vi "edit.vi"(8 "error in (no error)":errorcluster, 11 "BaseM1M3Settings in":refnum<class "M1M3Settings.lvclass">) -> (0 "error out":errorcluster, 2 "cancelIsTrue out":bool, 3 "BaseM1M3Settings out":refnum<class "M1M3Settings.lvclass">)   [LabVIEW 2016, in "M1M3Settings.lvclass"]
uses:
  M1M3Settings.lvclass
  D:/Code/ts_M1M3Support/Settings/Settings/Setting.lvclass
  DataTypes/Settings/Set/HPSettings.ctl
  Settings/Setting.lvclass/Setting.ctl
  <vilib>/Utility/xml.llb/Write to XML File(string).vi
  Settings/Setting.lvclass
  DataTypes/Settings/M1M3SupportSettings.lvlib
panel:
  in  "SettingTab":enum32{"HP Settings"}(tab)
  in  "HPSettings":T1
  in  "cancelIsTrue":bool
  out "String":string
  in  "saveIsTrue":bool
  in  "Listbox":i32(listbox)
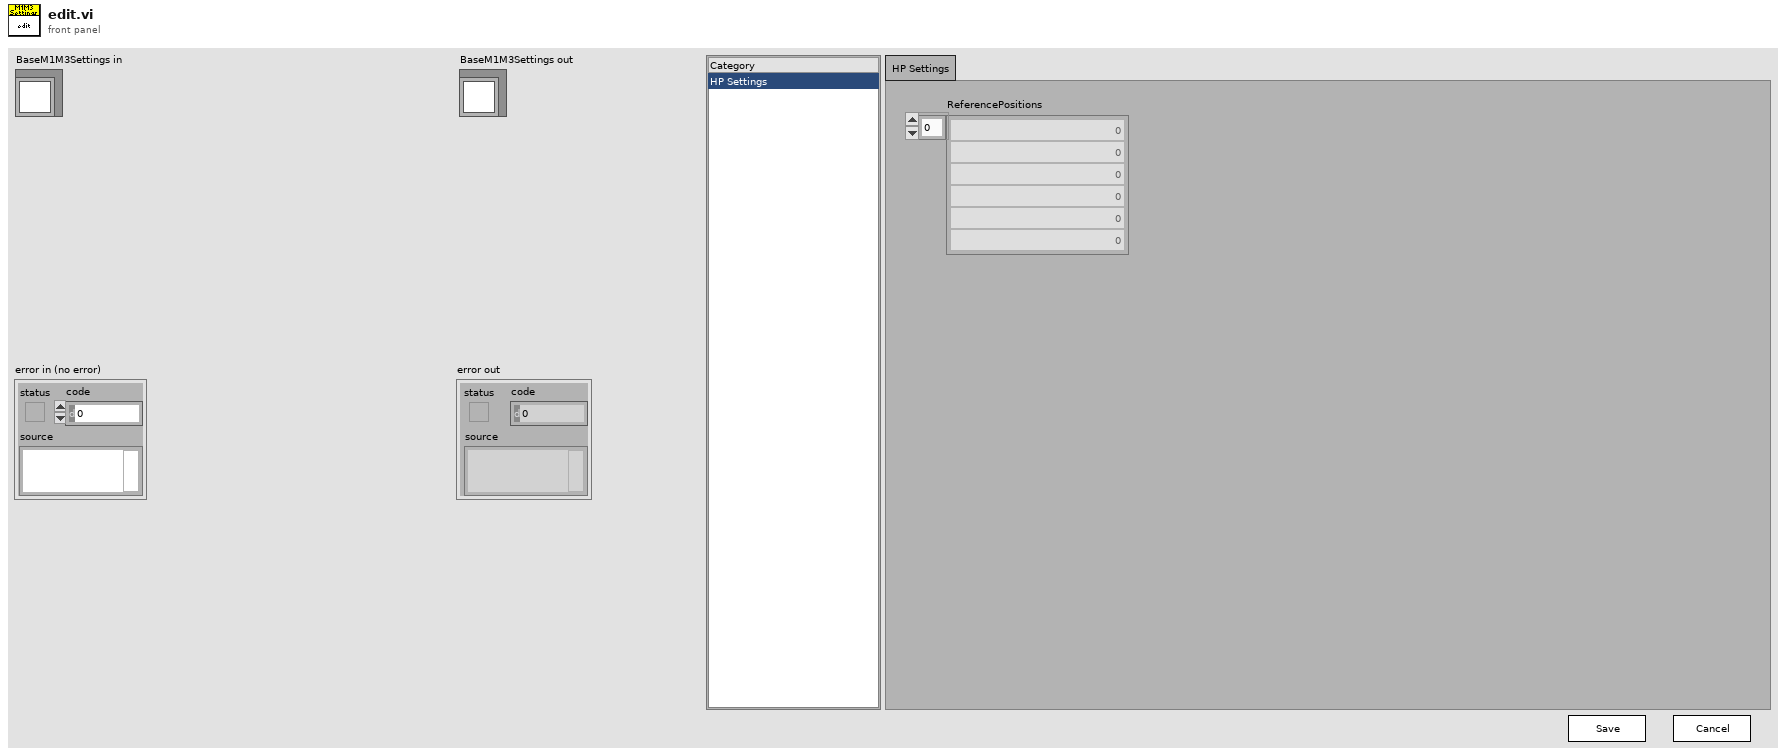
[diagram p1: front panel]
types:
  T1 = typedef "M1M3SupportSettings.lvlib/HPSettings.ctl" = cluster{"ReferencePositions":i32[]}
  T2 = enum16{"open", "replace", "create", "open or create", "replace or create", "replace or create with confirmation"}
  T3 = typedef "M1M3SupportTypes.lvlib/HPSettings.ctl" = cluster{"ReferencePositions":i32[]}
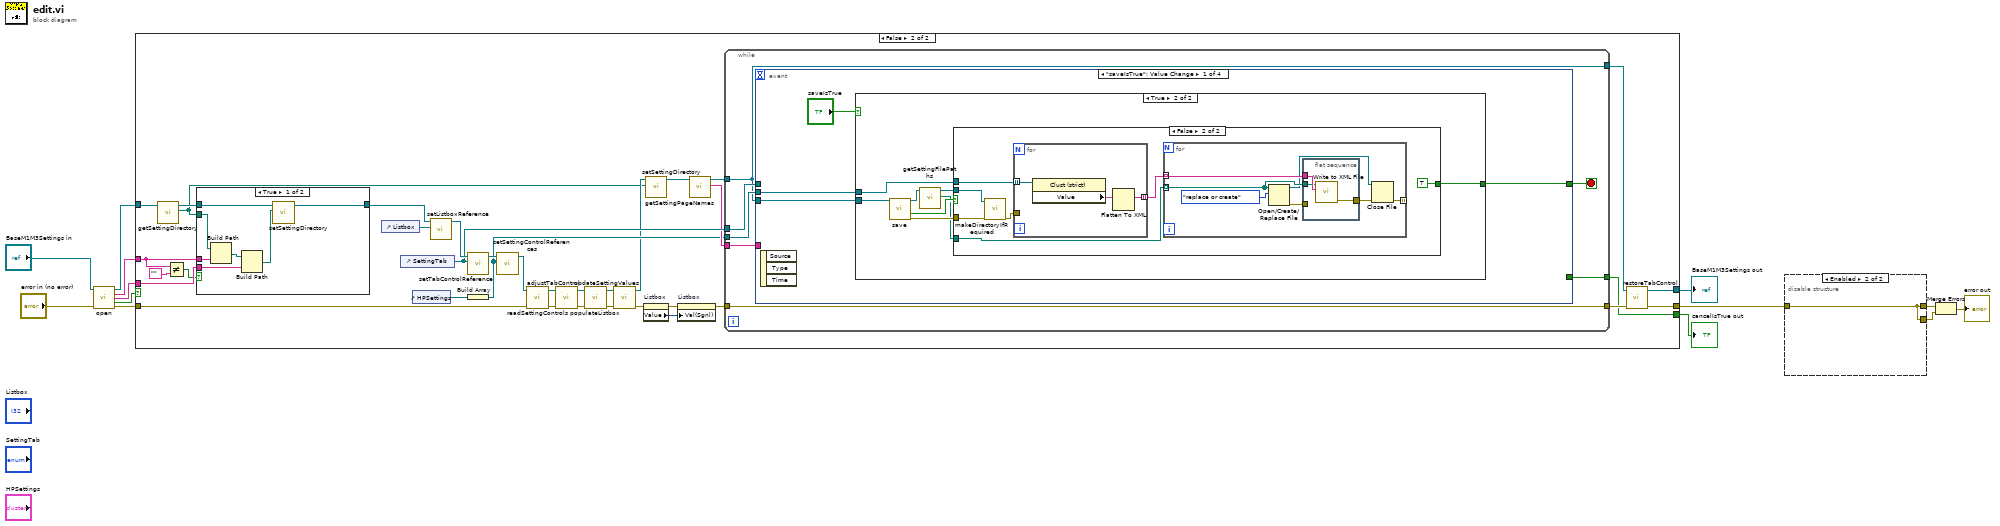
[diagram p0: block diagram]
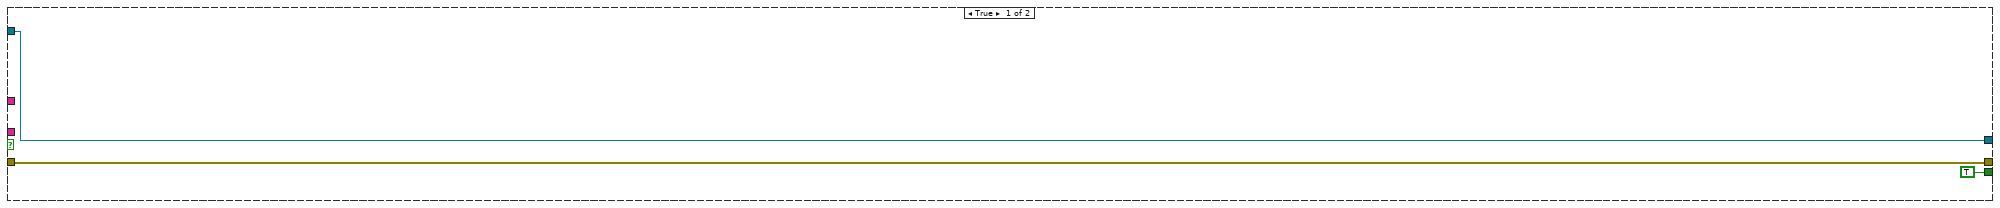
[diagram p2: hidden frame]
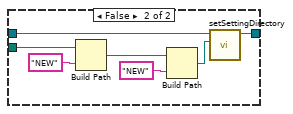
[diagram p3: hidden frame]
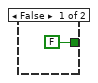
[diagram p4: hidden frame]
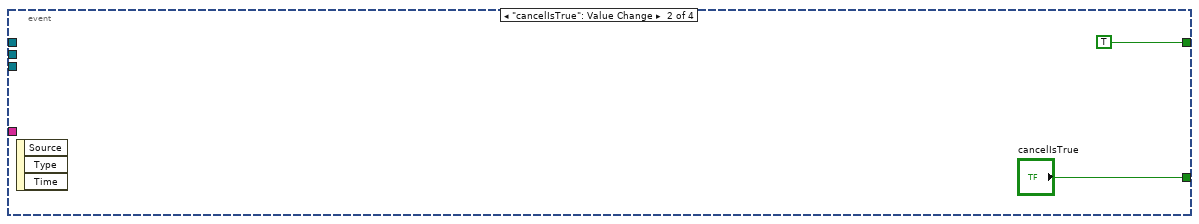
[diagram p6: hidden frame]
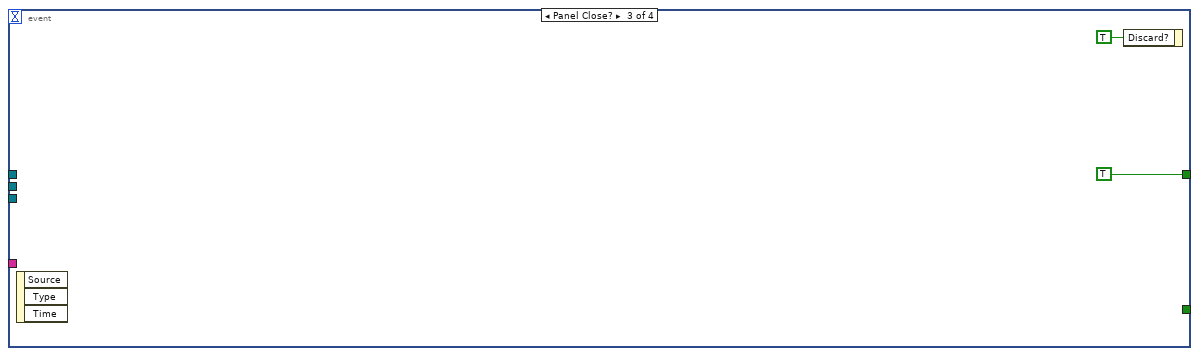
[diagram p7: hidden frame]
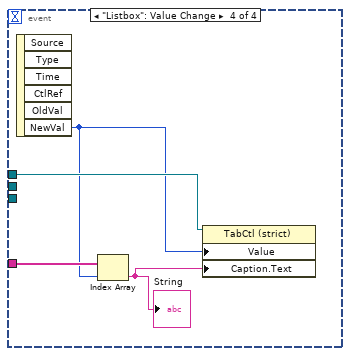
[diagram p8: hidden frame]
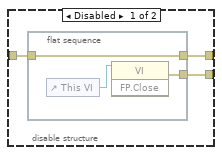
[diagram p9: hidden frame]
diagram:
  n1 = call "open.vi"("M1M3Settings in"="BaseM1M3Settings in", "error in (no error)"="error in (no error)") -> ("M1M3Settings out"=w12:refnum<class "M1M3Settings.lvclass">, "SelectedSet"=w3:string, "SelectedVersion"=w8:string, "Canceled"=w1:bool, "error out"=w4:errorcluster)  [unwired: 9 in]
  n2 = case shown="False" w1 {
    tunnel: w12 -> [w16 w43]
    tunnel: w8 -> [_ w27]
    tunnel: [w16 w26] -> w7
    tunnel: [w14 w25] -> w6
    tunnel: w4 -> [w14 w24]
    tunnel: w3 -> [_ w22]
    tunnel: [TRUE ("cancelIsTrue") w17] -> w2
    frame True {
    }
    frame False {
      n3 = call "getSettingDirectory.vi"("BaseSetting in"=w43) -> ("SettingDirectory"=w18:path, "BaseSetting out"=w42:refnum<class "M1M3Settings.lvclass">)  [unwired: 9 in]
      n4 = Not Equal?(x=w22, y="") -> (x != y?=w21:bool)
      n5 = case shown="True" w21 {
        tunnel: w42 -> [w58 w65]
        tunnel: [w57 w64] -> w28
        tunnel: w27 -> [w55 _]
        tunnel: w18 -> [w53 w61]
        tunnel: w22 -> [w52 _]
        frame True {
          n6 = Build Path(base path=w53, name or relative path=w52) -> (appended path=w56:path)
          n7 = Build Path(base path=w56, name or relative path=w55) -> (appended path=w54:path)
          n8 = call "setSettingDirectory.vi"("SettingDirectory"=w54, "BaseSetting in"=w58) -> ("BaseSetting out"=w57:refnum<class "M1M3Settings.lvclass">)  [unwired: 9 in]
        }
        frame False {
          n9 = Build Path(base path=w61, name or relative path="NEW") -> (appended path=w63:path)
          n10 = Build Path(base path=w63, name or relative path="NEW") -> (appended path=w62:path)
          n11 = call "setSettingDirectory.vi"("SettingDirectory"=w62, "BaseSetting in"=w65) -> ("BaseSetting out"=w64:refnum<class "M1M3Settings.lvclass">)  [unwired: 9 in]
        }
      }
      n12 = control-ref of="Listbox"() -> (w45:refnum<vi>)
      n13 = control-ref of="SettingTab"() -> (w35:refnum<vi>)
      n14 = control-ref of="HPSettings"() -> (w44:refnum<vi>)
      n15 = call "setListboxReference.vi"("ListboxReference"=w45, "Setting in"=w28) -> ("Setting out"=w46:refnum<class "M1M3Settings.lvclass">)  [unwired: 9 in]
      n16 = call "setTabControlReference.vi"("TabControlReference"=w35, "Setting in"=w46) -> ("Setting out"=w47:refnum<class "M1M3Settings.lvclass">)  [unwired: 9 in]
      n17 = Build Array(w44) -> (w32:refnum<vi>[])
      n18 = call "setSettingControlReferences.vi"("SettingControlReferences"=w32, "Setting in"=w47) -> ("Setting out"=w48:refnum<class "M1M3Settings.lvclass">)  [unwired: 9 in]
      n19 = call "readSettingControls.vi"("error in (no error)"=w24, "BaseSetting in"=w48) -> ("error out"=w38:errorcluster, "BaseSetting out"=w49:refnum<class "M1M3Settings.lvclass">)  [unwired: 8 in]
      n20 = call "adjustTabControl.vi"("error in (no error)"=w38, "BaseSetting in"=w49) -> ("error out"=w37:errorcluster, "BaseSetting out"=w50:refnum<class "M1M3Settings.lvclass">)  [unwired: 8 in]
      n21 = call "populateListbox.vi"("error in (no error)"=w37, "BaseSetting in"=w50) -> ("error out"=w36:errorcluster, "BaseSetting out"=w51:refnum<class "M1M3Settings.lvclass">)  [unwired: 8 in]
      n22 = call "updateSettingValues.vi"("error in (no error)"=w36, "BaseSetting in"=w51) -> ("error out"=w39:errorcluster, "BaseSetting out"=w20:refnum<class "M1M3Settings.lvclass">)  [unwired: 8 in]
      n23 = property on="Listbox" class="LstBox (strict)"(error in=w39) -> (error out=w41:errorcluster, "Value"=w40:i32)  [unwired: 1 in, 1 out]
      n24 = call "setSettingDirectory.vi"("SettingDirectory"=w18, "BaseSetting in"=w20) -> ("BaseSetting out"=w19:refnum<class "M1M3Settings.lvclass">)  [unwired: 9 in]
      n25 = property on="Listbox" class="LstBox (strict)"(error in=w41, "Val(Sgnl)"=w40) -> (error out=w31:errorcluster)  [unwired: 1 in, 1 out]
      n26 = call "getSettingPageNames.vi"("Setting in"=w19) -> ("SettingPageNames"=w33:string[], "Setting out"=w34:refnum<class "M1M3Settings.lvclass">)  [unwired: 9 in]
      n27 = while {
        tunnel: w35 -> [w70]
        tunnel: w32 -> [w72]
        tunnel: [w67] -> w29
        tunnel: w34 -> [w67]
        tunnel: w31 -> [w69]
        tunnel: [w69] -> w30
        tunnel: [w68] -> w17
        tunnel: w33 -> [w66]
        stop <- w71 stop-if-true
        n28 = event shown="[0] \"saveIsTrue\": Value Change" {
          selector: _ -> [_ _ _ _]
          dyn-events: _ -> [_ _ _ _]
          timeout: _ -> [_ _ _ _]
          tunnel: [w74 TRUE TRUE _] -> w71
          tunnel: w66 -> [_ _ _ w112]
          tunnel: w70 -> [_ _ _ w113]
          tunnel: w72 -> [w76 _ _ _]
          tunnel: [_ "cancelIsTrue" _ _] -> w68
          tunnel: w67 -> [w75 _ _ _]
          event "saveIsTrue": Value Change {
            n29 = event-data() -> ()  [unwired: 1 in, 3 out]
            n30 = case shown="True" "saveIsTrue" {
              tunnel: w76 -> [_ w85]
              tunnel: w75 -> [_ w84]
              tunnel: [FALSE w82] -> w74
              frame False {
              }
              frame True {
                n31 = call "save.vi"("M1M3Settings in"=w84) -> ("M1M3Settings out"=w80:refnum<class "M1M3Settings.lvclass">, "Canceled"=w81:bool, "error out"=w83:errorcluster)  [unwired: 12 in]
                n32 = call "getSettingFilePaths.vi"("Setting in"=w80) -> ("SettingFilePaths"=w78:path[], "Setting out"=w79:refnum<class "M1M3Settings.lvclass">)  [unwired: 9 in]
                n33 = case shown="False" w81 {
                  tunnel: w78 -> [_ w92]
                  tunnel: w85 -> [_ w91]
                  tunnel: w79 -> [_ w88]
                  tunnel: w83 -> [_ w87]
                  tunnel: [_ TRUE] -> w82
                  frame True {
                  }
                  frame False {
                    n34 = call "makeDirectoryIfRequired.vi"("error in (no error)"=w87, "BaseSetting in"=w88) -> ("error out"=w89:errorcluster)  [unwired: 8 in, 1 out]
                    n35 = for {
                      tunnel: w91 -> [w105] mode=indexing
                      tunnel: [w103] -> w90 mode=indexing
                      tunnel: w89 -> [_]
                      n36 = property class="Clust (strict)"(reference=w105) -> ("Value"=w104:T3)  [unwired: 1 in, 2 out]
                      n37 = Flatten To XML(anything=w104) -> (xml string=w103:string)
                    }
                    n38 = for {
                      tunnel: w92 -> [w96] mode=indexing
                      tunnel: w90 -> [w99] mode=indexing
                      tunnel: [w93] -> _ mode=indexing
                      n39 = Open/Create/Replace File(file path (use dialog)=w96, operation (0:open)=T2."replace or create") -> (refnum out=w95:refnum<file>, error out=w97:errorcluster)  [unwired: 4 in, 1 out]
                      n40 = flat-sequence {
                        tunnel: w99 -> [w102]
                        tunnel: [w101] -> w94
                        tunnel: w97 -> [_]
                        tunnel: w96 -> [w100]
                        frame #0 {
                          n41 = call-poly <vilib>:"Write to XML File.vi"("XML Input"=w102, "XML File Path"=w100) -> ("error out"=w101:errorcluster)  [unwired: 7 in, 2 out]
                        }
                      }
                      n42 = Close File(refnum=w95, error in=w94) -> (error out=w93:errorcluster)  [unwired: 1 out]
                    }
                  }
                }
              }
            }
          }
          event "cancelIsTrue": Value Change {
            n43 = event-data() -> ()  [unwired: 1 in, 3 out]
          }
          event Panel Close? {
            n44 = event-data() -> ()  [unwired: 1 in, 3 out]
            n45 = event-data("Discard?"=TRUE) -> ()  [unwired: 1 in, 1 out]
          }
          event "Listbox": Value Change {
            n46 = event-data() -> ("NewVal"=w111:i32)  [unwired: 1 in, 5 out]
            n47 = Index Array(array=w112, index=w111) -> (element=w110:string)
            "String" <- w110
            n48 = property class="TabCtl (strict)"(reference=w113, "Value"=w111, "Caption.Text"=w110) -> ()  [unwired: 1 in, 2 out]
          }
        }
      }
      n49 = call "restoreTabControl.vi"("error in (no error)"=w30, "BaseSetting in"=w29) -> ("error out"=w25:errorcluster, "BaseSetting out"=w26:refnum<class "M1M3Settings.lvclass">)  [unwired: 8 in]
    }
  }
  "BaseM1M3Settings out" <- w7
  "cancelIsTrue out" <- w2
  n50 = disable-structure shown="Enabled" {
    disable-tunnel: [w116 w120] -> w11
    disable-tunnel: [w115 w120] -> w10
    disable-tunnel: w6 -> [w114 w120]
    frame Disabled {
      n51 = flat-sequence {
        tunnel: [w118] -> w116
        tunnel: [w117] -> w115
        tunnel: w114 -> [w117]
        frame #0 {
          n52 = control-ref of="This VI"() -> (w119:refnum<vi>)
          n53 = invoke class="VI" method="FP.Close"(reference=w119) -> (error out=w118:errorcluster)  [unwired: 2 in, 2 out]
        }
      }
    }
    frame Enabled {
    }
  }
  n54 = Merge Errors(w10, w11) -> (→"error out":errorcluster)
